vi "Get Data.vi"(8 "error in (no error)":errorcluster, 11 "Number in":refnum<class "Number.lvclass">) -> (0 "error out":errorcluster, 3 "Number out":refnum<class "Number.lvclass">)   [LabVIEW 2023, in "Number.lvclass"]
uses:
  Number.lvclass
  Number.lvclass/Number.ctl
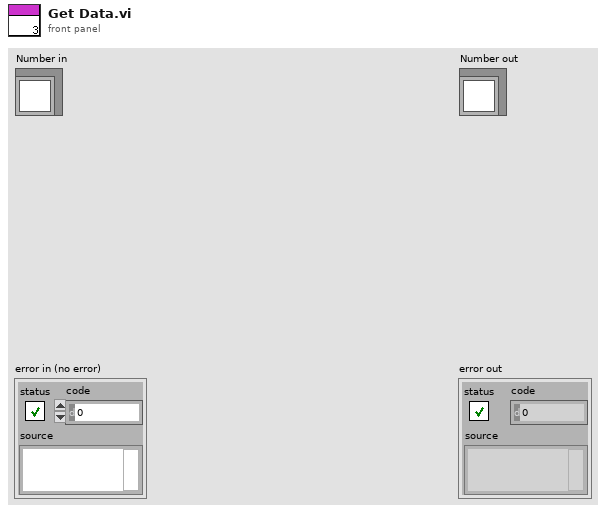
[diagram p1: front panel]
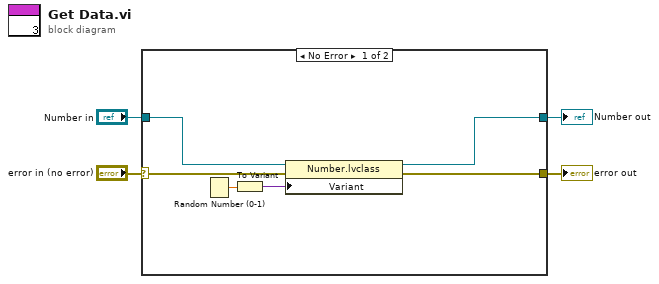
[diagram p0: block diagram]
diagram:
  n1 = case shown="No Error" "error in (no error)" {
    selector: "error in (no error)" -> [w10 w12]
    tunnel: [w9 w12] -> w3
    tunnel: [w7 w11] -> w1
    tunnel: "Number in" -> [w8 w11]
    frame No Error {
      n2 = Random Number (0-1)() -> (number: 0 to 1=w6:dbl)
      n3 = To Variant(anything=w6) -> (Variant=w5:variant)
      n4 = property class="Number.lvclass"(reference=w8, error in=w10, "Variant"=w5) -> (reference out=w7:refnum<class "Number.lvclass">, error out=w9:errorcluster)
    }
    frame Error {
    }
  }
  "error out" <- w3
  "Number out" <- w1
